vi "LaserQuantum_Settings.vi"(8 "error in (no error)":errorcluster, 10 "Timeout":u32=100, 11 "COM port":refnum<visa-resource-name>) -> (0 "error out":errorcluster)   [LabVIEW 2018]
panel:
  out "PSU temperature":dbl
  out "Laser temperature":dbl
  in  "Laser on":bool
  in  "OK Button":bool
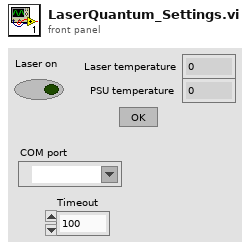
[diagram p1: front panel]
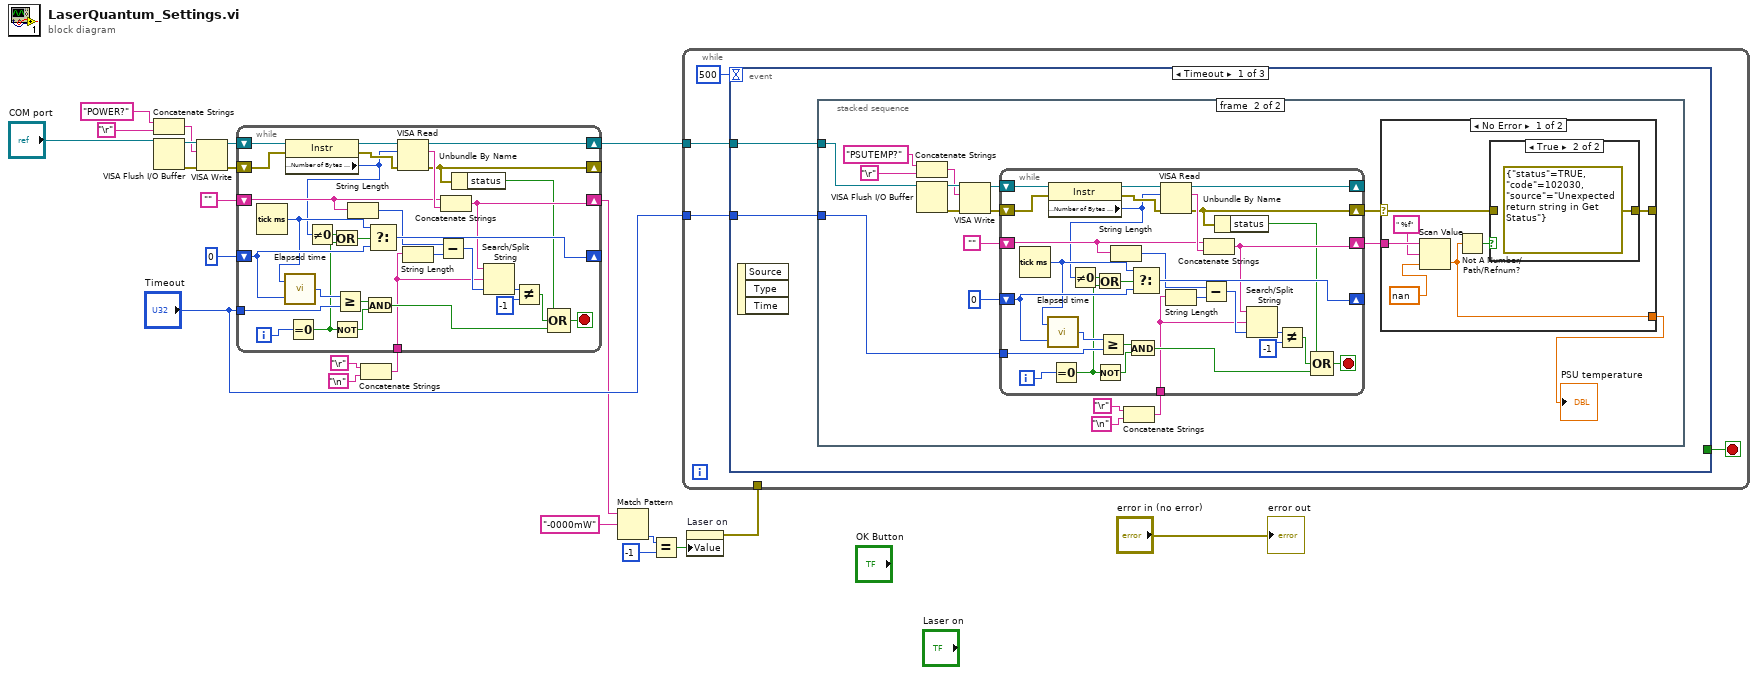
[diagram p0: block diagram]
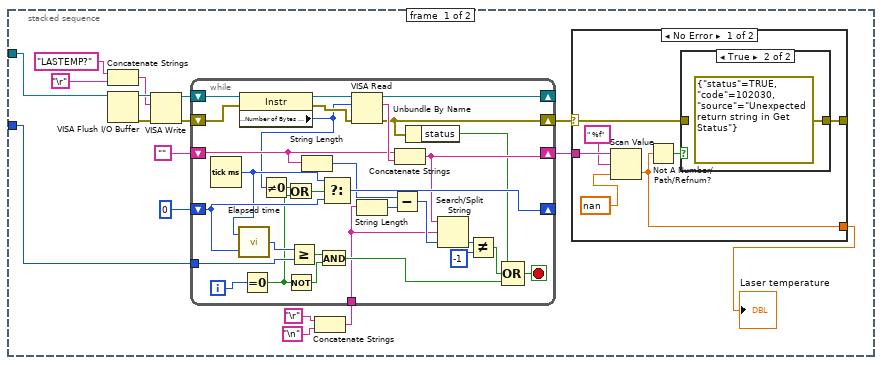
[diagram p2: hidden frame]
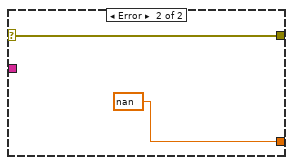
[diagram p4: hidden frame]
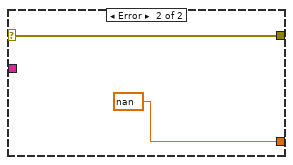
[diagram p6: hidden frame]
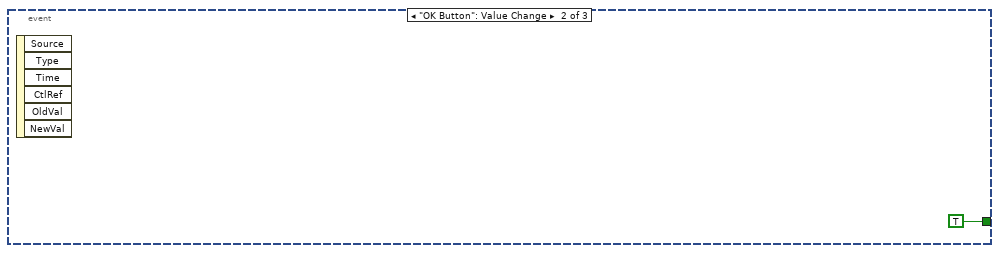
[diagram p7: hidden frame]
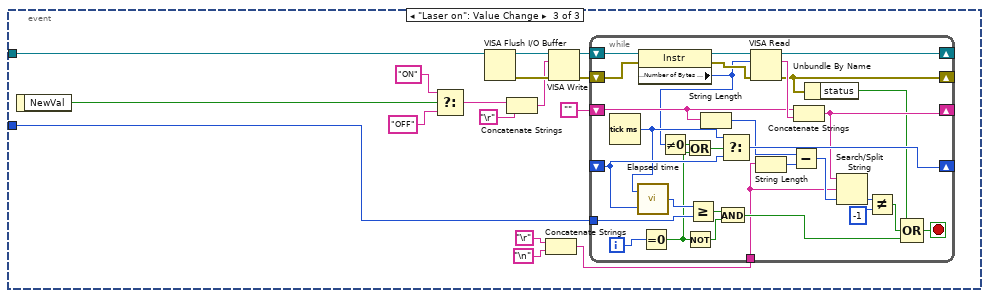
[diagram p8: hidden frame]
diagram:
  n1 = Concatenate Strings("POWER?", "\r") -> (w11:string)
  n2 = VISA Flush I/O Buffer(VISA resource name="COM port") -> (VISA resource name out=w21:refnum<visa-resource-name>, error out=w20:errorcluster)  [unwired: 2 in]
  n3 = VISA Write(VISA resource name=w21, write buffer=w11, error in (no error)=w20) -> (VISA resource name out=w19:refnum<visa-resource-name>, error out=w18:errorcluster)  [unwired: 1 out]
  n4 = Concatenate Strings("\r", "\n") -> (w13:string)
  n5 = while {
    shift-right: [w49] -> w9
    shift-left: w19 -> [w53]
    shift-right: [w25] -> _
    shift-left: w18 -> [w52]
    shift-right: [w32] -> w6
    shift-left: "" -> [w31]
    shift-right: [w40] -> _
    shift-left: u32 0 -> [w37]
    tunnel: "Timeout" -> [w38]
    tunnel: w13 -> [w26]
    i -> [w42]
    stop <- w48 stop-if-true
    n6 = Tick Count (ms)() -> (millisecond timer value=w24:u32)
    n7 = call "Elapsed time.vi"("Start time (ms)"=w37, "Current time (ms)"=w24) -> ("Elapsed time"=w39:u32)
    n8 = property class="Instr"(reference=w53, error in=w52) -> (reference out=w51:refnum<visa-resource-name>, error out=w50:errorcluster, "Serial Settings:Number of Bytes at Serial Port"=w23:u32)
    n9 = Equal To 0?(x=w42) -> (x = 0?=w33:bool)
    n10 = Not Equal To 0?(x=w23) -> (x != 0?=w43:bool)
    n11 = Or(x=w43, y=w33) -> (x .or. y?=w41:bool)
    n12 = Not(x=w33) -> (.not. x?=w34:bool)
    n13 = Greater Or Equal?(x=w39, y=w38) -> (x >= y?=w35:bool)
    n14 = String Length(string=w31) -> (length=w29:i32)
    n15 = And(x=w35, y=w34) -> (x .and. y?=w36:bool)
    n16 = Select(t=w24, s=w41, f=w37) -> (s? t:f=w40:u32)
    n17 = VISA Read(VISA resource name=w51, byte count=w23, error in (no error)=w50) -> (VISA resource name out=w49:refnum<visa-resource-name>, read buffer=w47:string, error out=w25:errorcluster)  [unwired: 1 out]
    n18 = String Length(string=w26) -> (length=w30:i32)
    n19 = Subtract(x=w29, y=w30) -> (x-y=w28:i32)
    n20 = Concatenate Strings(w31, w47) -> (w32:string)
    n21 = Unbundle By Name(w25) -> ("status"=w27:bool)
    n22 = Search/Split String(string=w32, search string/char (-)=w26, offset (0)=w28) -> (offset of match=w46:i32)  [unwired: 2 out]
    n23 = Not Equal?(x=w46, y=-1) -> (x != y?=w44:bool)
    n24 = Compound Arithmetic op=OR(w27, w44, w36) -> (w48:bool)
  }
  n25 = Match Pattern(string=w6, regular expression="-0000mW") -> (offset past match=w4:i32)  [unwired: 1 in, 3 out]
  n26 = Equal?(x=w4, y=-1) -> (x = y?=w2:bool)
  n27 = property on="Laser on" class="Bool (strict)"("Value"=w2) -> (error out=w1:errorcluster)  [unwired: 2 in, 1 out]
  n28 = while {
    tunnel: w9 -> [w56]
    tunnel: "Timeout" -> [w55]
    tunnel: w1 -> [_]
    stop <- w57 stop-if-true
    n29 = event shown="[0] Timeout" {
      selector: _ -> [_ _ _]
      dyn-events: _ -> [_ _ _]
      timeout: 500 -> [_ _ _]
      tunnel: [_ TRUE _] -> w57
      tunnel: w56 -> [w59 _ w184]
      tunnel: w55 -> [w58 _ w183]
      event Timeout {
        n30 = event-data() -> ()  [unwired: 1 in, 3 out]
        n31 = stacked-sequence {
          tunnel: w59 -> [w61 w120]
          tunnel: w58 -> [w60 w119]
          frame #0 {
            n32 = Concatenate Strings("LASTEMP?", "\r") -> (w66:string)
            n33 = VISA Flush I/O Buffer(VISA resource name=w61) -> (VISA resource name out=w76:refnum<visa-resource-name>, error out=w75:errorcluster)  [unwired: 2 in]
            n34 = VISA Write(VISA resource name=w76, write buffer=w66, error in (no error)=w75) -> (VISA resource name out=w74:refnum<visa-resource-name>, error out=w73:errorcluster)  [unwired: 1 out]
            n35 = Concatenate Strings("\r", "\n") -> (w68:string)
            n36 = while {
              shift-right: [w114] -> _
              shift-left: w74 -> [w118]
              shift-right: [w90] -> w64
              shift-left: w73 -> [w117]
              shift-right: [w97] -> w63
              shift-left: "" -> [w96]
              shift-right: [w105] -> _
              shift-left: u32 0 -> [w102]
              tunnel: w60 -> [w103]
              tunnel: w68 -> [w91]
              i -> [w107]
              stop <- w113 stop-if-true
              n37 = Tick Count (ms)() -> (millisecond timer value=w89:u32)
              n38 = call "Elapsed time.vi"("Start time (ms)"=w102, "Current time (ms)"=w89) -> ("Elapsed time"=w104:u32)
              n39 = property class="Instr"(reference=w118, error in=w117) -> (reference out=w116:refnum<visa-resource-name>, error out=w115:errorcluster, "Serial Settings:Number of Bytes at Serial Port"=w88:u32)
              n40 = Equal To 0?(x=w107) -> (x = 0?=w98:bool)
              n41 = Not Equal To 0?(x=w88) -> (x != 0?=w108:bool)
              n42 = Or(x=w108, y=w98) -> (x .or. y?=w106:bool)
              n43 = Not(x=w98) -> (.not. x?=w99:bool)
              n44 = Greater Or Equal?(x=w104, y=w103) -> (x >= y?=w100:bool)
              n45 = String Length(string=w96) -> (length=w94:i32)
              n46 = And(x=w100, y=w99) -> (x .and. y?=w101:bool)
              n47 = Select(t=w89, s=w106, f=w102) -> (s? t:f=w105:u32)
              n48 = VISA Read(VISA resource name=w116, byte count=w88, error in (no error)=w115) -> (VISA resource name out=w114:refnum<visa-resource-name>, read buffer=w112:string, error out=w90:errorcluster)  [unwired: 1 out]
              n49 = String Length(string=w91) -> (length=w95:i32)
              n50 = Subtract(x=w94, y=w95) -> (x-y=w93:i32)
              n51 = Concatenate Strings(w96, w112) -> (w97:string)
              n52 = Unbundle By Name(w90) -> ("status"=w92:bool)
              n53 = Search/Split String(string=w97, search string/char (-)=w91, offset (0)=w93) -> (offset of match=w111:i32)  [unwired: 2 out]
              n54 = Not Equal?(x=w111, y=-1) -> (x != y?=w109:bool)
              n55 = Compound Arithmetic op=OR(w92, w109, w101) -> (w113:bool)
            }
            n56 = case shown="No Error" w64 {
              selector: w64 -> [w82 w87]
              tunnel: w63 -> [w80 _]
              tunnel: [w83 w87] -> _
              tunnel: [w77 nan] -> w62
              frame No Error {
                n57 = Scan Value(string=w80, format string=" %f", default (0 dbl)=nan ("t")) -> (value=w77:dbl)  [unwired: 1 out]
                n58 = Not A Number/Path/Refnum?(number/path/refnum=w77) -> (NaN/Path/Refnum?=w81:bool)
                n59 = case shown="True" w81 {
                  tunnel: [w84 errorcluster {"status"=TRUE, "code"=102030, "source"="Unexpected return string in Get Status"} ("error IO")] -> w83
                  tunnel: w82 -> [w84 _]
                  frame False {
                  }
                  frame True {
                  }
                }
              }
              frame Error {
              }
            }
            "Laser temperature" <- w62
          }
          frame #1 {
            n60 = Concatenate Strings("PSUTEMP?", "\r") -> (w125:string)
            n61 = VISA Flush I/O Buffer(VISA resource name=w120) -> (VISA resource name out=w135:refnum<visa-resource-name>, error out=w134:errorcluster)  [unwired: 2 in]
            n62 = VISA Write(VISA resource name=w135, write buffer=w125, error in (no error)=w134) -> (VISA resource name out=w133:refnum<visa-resource-name>, error out=w132:errorcluster)  [unwired: 1 out]
            n63 = Concatenate Strings("\r", "\n") -> (w127:string)
            n64 = while {
              shift-right: [w173] -> _
              shift-left: w133 -> [w177]
              shift-right: [w149] -> w123
              shift-left: w132 -> [w176]
              shift-right: [w156] -> w122
              shift-left: "" -> [w155]
              shift-right: [w164] -> _
              shift-left: u32 0 -> [w161]
              tunnel: w119 -> [w162]
              tunnel: w127 -> [w150]
              i -> [w166]
              stop <- w172 stop-if-true
              n65 = Tick Count (ms)() -> (millisecond timer value=w148:u32)
              n66 = call "Elapsed time.vi"("Start time (ms)"=w161, "Current time (ms)"=w148) -> ("Elapsed time"=w163:u32)
              n67 = property class="Instr"(reference=w177, error in=w176) -> (reference out=w175:refnum<visa-resource-name>, error out=w174:errorcluster, "Serial Settings:Number of Bytes at Serial Port"=w147:u32)
              n68 = Equal To 0?(x=w166) -> (x = 0?=w157:bool)
              n69 = Not Equal To 0?(x=w147) -> (x != 0?=w167:bool)
              n70 = Or(x=w167, y=w157) -> (x .or. y?=w165:bool)
              n71 = Not(x=w157) -> (.not. x?=w158:bool)
              n72 = Greater Or Equal?(x=w163, y=w162) -> (x >= y?=w159:bool)
              n73 = String Length(string=w155) -> (length=w153:i32)
              n74 = And(x=w159, y=w158) -> (x .and. y?=w160:bool)
              n75 = Select(t=w148, s=w165, f=w161) -> (s? t:f=w164:u32)
              n76 = VISA Read(VISA resource name=w175, byte count=w147, error in (no error)=w174) -> (VISA resource name out=w173:refnum<visa-resource-name>, read buffer=w171:string, error out=w149:errorcluster)  [unwired: 1 out]
              n77 = String Length(string=w150) -> (length=w154:i32)
              n78 = Subtract(x=w153, y=w154) -> (x-y=w152:i32)
              n79 = Concatenate Strings(w155, w171) -> (w156:string)
              n80 = Unbundle By Name(w149) -> ("status"=w151:bool)
              n81 = Search/Split String(string=w156, search string/char (-)=w150, offset (0)=w152) -> (offset of match=w170:i32)  [unwired: 2 out]
              n82 = Not Equal?(x=w170, y=-1) -> (x != y?=w168:bool)
              n83 = Compound Arithmetic op=OR(w151, w168, w160) -> (w172:bool)
            }
            n84 = case shown="No Error" w123 {
              selector: w123 -> [w141 w146]
              tunnel: w122 -> [w139 _]
              tunnel: [w142 w146] -> _
              tunnel: [w136 nan] -> w121
              frame No Error {
                n85 = Scan Value(string=w139, format string=" %f", default (0 dbl)=nan ("t")) -> (value=w136:dbl)  [unwired: 1 out]
                n86 = Not A Number/Path/Refnum?(number/path/refnum=w136) -> (NaN/Path/Refnum?=w140:bool)
                n87 = case shown="True" w140 {
                  tunnel: [w143 errorcluster {"status"=TRUE, "code"=102030, "source"="Unexpected return string in Get Status"} ("error IO")] -> w142
                  tunnel: w141 -> [w143 _]
                  frame False {
                  }
                  frame True {
                  }
                }
              }
              frame Error {
              }
            }
            "PSU temperature" <- w121
          }
        }
      }
      event "OK Button": Value Change {
        n88 = event-data() -> ()  [unwired: 1 in, 6 out]
      }
      event "Laser on": Value Change {
        n89 = event-data() -> ("NewVal"=w182:bool)  [unwired: 1 in]
        n90 = Select(t="ON", s=w182, f="OFF") -> (s? t:f=w179:string)
        n91 = VISA Flush I/O Buffer(VISA resource name=w184) -> (VISA resource name out=w190:refnum<visa-resource-name>, error out=w192:errorcluster)  [unwired: 2 in]
        n92 = Concatenate Strings(w179, "\r") -> (w191:string)
        n93 = Concatenate Strings("\r", "\n") -> (w189:string)
        n94 = VISA Write(VISA resource name=w190, write buffer=w191, error in (no error)=w192) -> (VISA resource name out=w193:refnum<visa-resource-name>, error out=w194:errorcluster)  [unwired: 1 out]
        n95 = while {
          shift-right: [w221] -> _
          shift-left: w193 -> [w225]
          shift-right: [w197] -> _
          shift-left: w194 -> [w224]
          shift-right: [w204] -> _
          shift-left: "" -> [w203]
          shift-right: [w212] -> _
          shift-left: _ -> [w209]
          tunnel: w183 -> [w210]
          tunnel: w189 -> [w198]
          i -> [w214]
          stop <- w220 stop-if-true
          n96 = Tick Count (ms)() -> (millisecond timer value=w196:u32)
          n97 = call "Elapsed time.vi"("Start time (ms)"=w209, "Current time (ms)"=w196) -> ("Elapsed time"=w211:u32)
          n98 = property class="Instr"(reference=w225, error in=w224) -> (reference out=w223:refnum<visa-resource-name>, error out=w222:errorcluster, "Serial Settings:Number of Bytes at Serial Port"=w195:u32)
          n99 = Equal To 0?(x=w214) -> (x = 0?=w205:bool)
          n100 = Not Equal To 0?(x=w195) -> (x != 0?=w215:bool)
          n101 = Or(x=w215, y=w205) -> (x .or. y?=w213:bool)
          n102 = Not(x=w205) -> (.not. x?=w206:bool)
          n103 = Greater Or Equal?(x=w211, y=w210) -> (x >= y?=w207:bool)
          n104 = String Length(string=w203) -> (length=w201:i32)
          n105 = And(x=w207, y=w206) -> (x .and. y?=w208:bool)
          n106 = Select(t=w196, s=w213, f=w209) -> (s? t:f=w212:u32)
          n107 = VISA Read(VISA resource name=w223, byte count=w195, error in (no error)=w222) -> (VISA resource name out=w221:refnum<visa-resource-name>, read buffer=w219:string, error out=w197:errorcluster)  [unwired: 1 out]
          n108 = String Length(string=w198) -> (length=w202:i32)
          n109 = Subtract(x=w201, y=w202) -> (x-y=w200:i32)
          n110 = Concatenate Strings(w203, w219) -> (w204:string)
          n111 = Unbundle By Name(w197) -> ("status"=w199:bool)
          n112 = Search/Split String(string=w204, search string/char (-)=w198, offset (0)=w200) -> (offset of match=w218:i32)  [unwired: 2 out]
          n113 = Not Equal?(x=w218, y=-1) -> (x != y?=w216:bool)
          n114 = Compound Arithmetic op=OR(w199, w216, w208) -> (w220:bool)
        }
      }
    }
  }
  "error out" <- "error in (no error)"
